vi "stageTriggerOutputTest.vi"() -> ()   [LabVIEW 2015]
panel:
  in  "Radio Buttons":enum32{"stop/ start", "cont."}(radio)
  in  "initPos (mm)":string="10"
  out "error out":errorcluster
  in  "finPos (mm)":string="10"
  in  "stepSize (mm)":string="1"
  in  "triggerOutputIdx":string="1"
  in  "Z stage":T1={"System no."=2, "zIdx"=1, "zLim (mm)"=13.0, "0, 1"=0} {"System no." min=1 step=1}
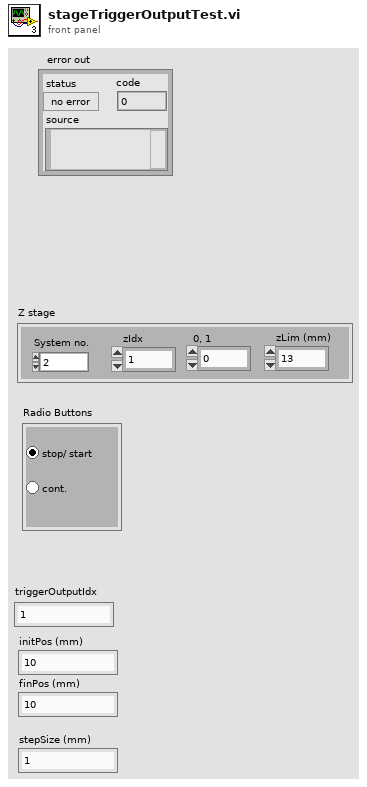
[diagram p1: front panel]
types:
  T1 = cluster{"System no.":i32, "zIdx":i32, "zLim (mm)":dbl, "0, 1":i16}
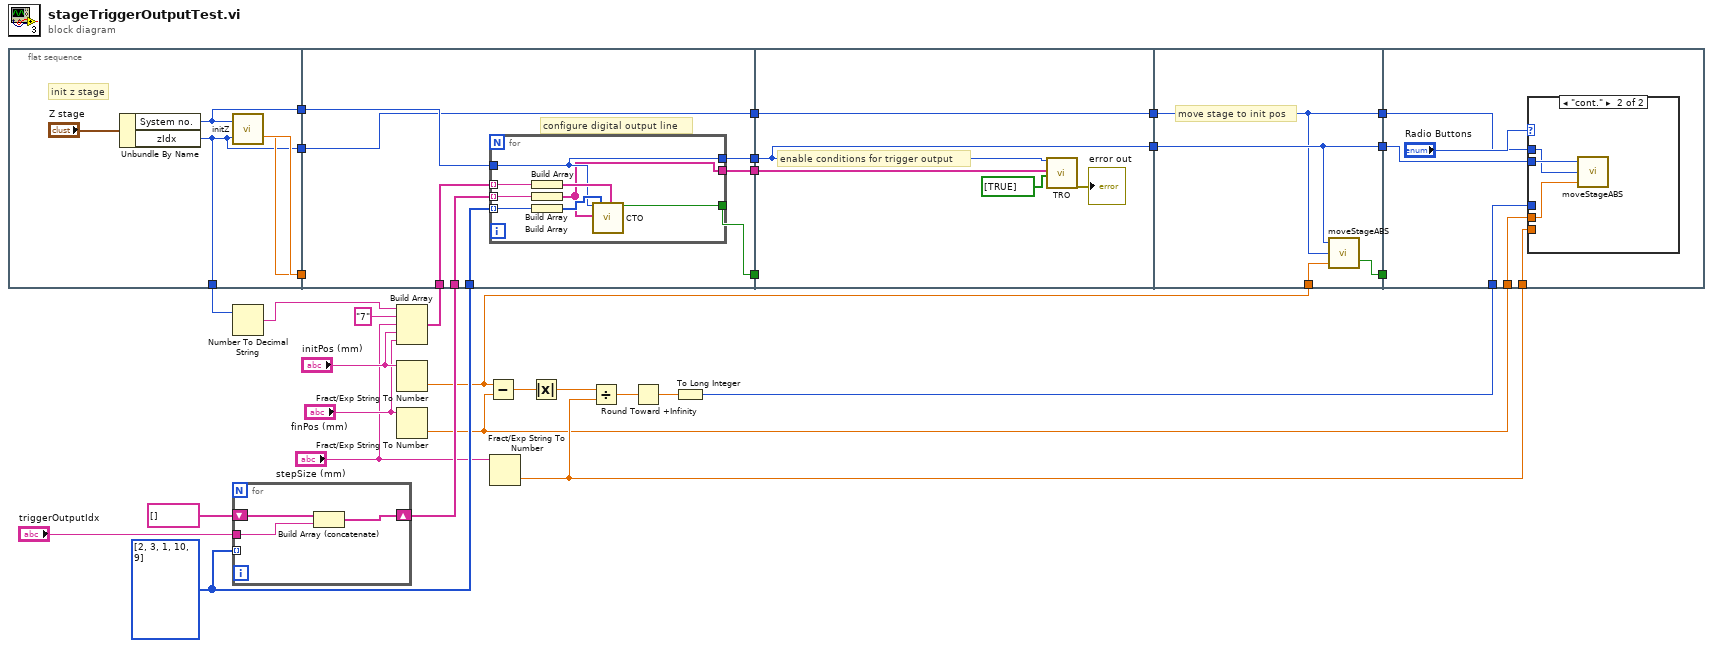
[diagram p0: block diagram]
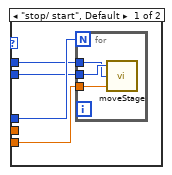
[diagram p2: hidden frame]
diagram:
  w27 = i32[] [2, 3, 1, 10, 9] ("CTO parameter ID")
  n1 = flat-sequence {
    tunnel: [w36] -> w32
    tunnel: [w35] -> w31
    tunnel: [w33] -> w26
    tunnel: [w34] -> w22
    tunnel: [w33] -> w17
    tunnel: w32 -> [_]
    tunnel: w31 -> [_]
    tunnel: w28 -> [w45]
    tunnel: w27 -> [w44]
    tunnel: w23 -> [w43]
    tunnel: w22 -> [w42]
    tunnel: [w41] -> w21
    tunnel: [w40] -> w20
    tunnel: [w39] -> w19
    tunnel: w17 -> [w38]
    tunnel: [w38] -> w16
    tunnel: w21 -> [_]
    tunnel: w20 -> [w55]
    tunnel: w19 -> [w58]
    tunnel: [w55] -> w18
    tunnel: w16 -> [w54]
    tunnel: [w54] -> w15
    tunnel: w18 -> [w60]
    tunnel: w15 -> [w59]
    tunnel: w8 -> [w62]
    tunnel: [w61] -> w6
    tunnel: [w60] -> w4
    tunnel: [w59] -> w3
    tunnel: w6 -> [_]
    tunnel: w5 -> [w67]
    tunnel: w4 -> [w66]
    tunnel: w3 -> [w65]
    tunnel: w2 -> [w64]
    tunnel: w1 -> [w63]
    frame #0 {
      # "init z stage"
      n2 = Unbundle By Name("Z stage") -> ("System no."=w34:i32, "zIdx"=w33:i32)
      n3 = call "initZ.vi"("zIdx"=w33, "System no."=w34) -> ("zLim"=w35:dbl, "zPos"=w36:dbl)
    }
    frame #1 {
      # "configure digital output line"
      n4 = for {
        tunnel: w45 -> [w52] mode=indexing
        tunnel: w44 -> [w53] mode=indexing
        tunnel: w43 -> [w51] mode=indexing
        tunnel: w42 -> [w47]
        tunnel: [w48] -> w41
        tunnel: [w47] -> w40
        tunnel: [w46] -> w39
        n5 = Build Array(w51) -> (w49:string[])
        n6 = Build Array(w52) -> (w46:string[])
        n7 = Build Array(w53) -> (w50:i32[])
        n8 = call "CTO.vi"("System no."=w47, "TriggerOut to set"=w46, "CTO parameter ID"=w50, "Parameter value"=w49) -> ("Controller error"=w48:bool)  [unwired: 14 in, 1 out]
      }
    }
    frame #2 {
      # "enable conditions for trigger output"
      n9 = call "TRO.vi"("System no."=w55, "TriggerOut to command"=w58, "Trigger status"=bool[] [TRUE]) -> ("error out"=→"error out":errorcluster)  [unwired: 16 in]
    }
    frame #3 {
      # "move stage to init pos"
      n10 = call "moveStageABS.vi"("absolute pos (mm)"=w62, "axisIdx"=w59, "System no."=w60) -> ("Stopped"=w61:bool)
    }
    frame #4 {
      n11 = case shown="\"cont.\"" "Radio Buttons" {
        tunnel: w67 -> [w72 _]
        tunnel: w66 -> [w71 w78]
        tunnel: w65 -> [w70 w77]
        tunnel: w64 -> [w69 _]
        tunnel: w63 -> [_ w76]
        frame "stop/ start", Default {
          n12 = for {
            N: w72 -> [_]
            tunnel: w71 -> [w75]
            tunnel: w70 -> [w74]
            tunnel: w69 -> [w73]
            n13 = call "moveStage.vi"("inc (mm)"=w73, "axisIdx"=w74, "System no."=w75) -> ()  [unwired: 1 out]
          }
        }
        frame "cont." {
          n14 = call "moveStageABS.vi"("absolute pos (mm)"=w76, "axisIdx"=w77, "System no."=w78) -> ()  [unwired: 1 out]
        }
      }
    }
  }
  n15 = Number To Decimal String(number=w26) -> (decimal integer string=w25:string)  [unwired: 1 in]
  n16 = for {
    shift-right: [w79] -> w28
    shift-left: string[] [] -> [w81]
    tunnel: "triggerOutputIdx" -> [w80]
    tunnel: w27 -> [_] mode=indexing
    n17 = Build Array (concatenate)(w81, w80) -> (w79:string[])
  }
  n18 = Build Array(w25, "7" ("element"), "stepSize (mm)", "initPos (mm)", "finPos (mm)") -> (w23:string[])
  n19 = Fract/Exp String To Number(string="initPos (mm)") -> (number=w8:dbl)  [unwired: 3 in, 1 out]
  n20 = Fract/Exp String To Number(string="finPos (mm)") -> (number=w1:dbl)  [unwired: 3 in, 1 out]
  n21 = Subtract(x=w8, y=w1) -> (x-y=w9:dbl)
  n22 = Fract/Exp String To Number(string="stepSize (mm)") -> (number=w2:dbl)  [unwired: 3 in, 1 out]
  n23 = Absolute Value(x=w9) -> (abs(x)=w10:dbl)
  n24 = Divide(x=w10, y=w2) -> (x/y=w11:dbl)
  n25 = Round Toward +Infinity(x=w11) -> (ceil(x): smallest int >= x=w12:dbl)
  n26 = To Long Integer(number=w12) -> (32bit integer=w5:i32)
